vi "Add ItemIDs.vi"(8 "error in":errorcluster, 11 "Panel in":refnum<class "Panel.lvclass">) -> (0 "error out":errorcluster, 3 "Panel out":refnum<class "Panel.lvclass">)   [LabVIEW 2021]
uses:
  <vilib>/OPCUA/controls/Data Type.ctl
  <vilib>/OPCUA/NI OPC UA Server.lvlib
  Panel.lvclass
  C:/GitHub/SM EOL OPC Server AF/Station/Station Actor/Station.lvclass
  C:/Program Files/National Instruments/LabVIEW 2021/vi.lib/ActorFramework/Actor/Actor.lvclass
  C:/GitHub/SM EOL OPC Server AF/Station Panel/Station Panel Actor/Panel.lvclass
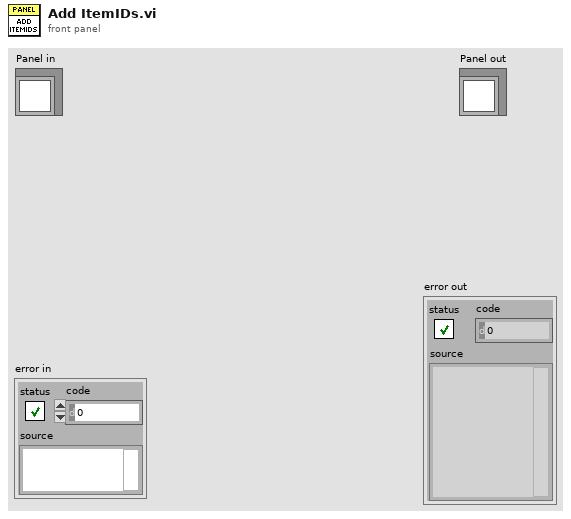
[diagram p1: front panel]
types:
  T1 = typedef "Data Type.ctl" = u16
  T2 = cluster{"name":string, "data type":T1, "access level":u16, "description":string}
  T3 = typedef "NodeId.ctl" = string
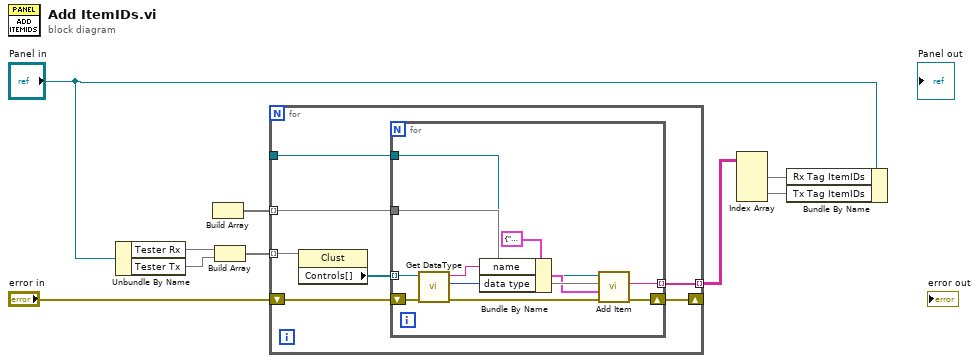
[diagram p0: block diagram]
diagram:
  n1 = Unbundle By Name("Panel in") -> ("Tester Rx"=w9, "Tester Tx"=w8)
  n2 = Build Array() -> (w2:void[])  [unwired: 2 in]
  n3 = Build Array(w9, w8) -> (w7:void[])
  n4 = for {
    tunnel: w7 -> [w14] mode=indexing
    tunnel: w2 -> [w13] mode=indexing
    tunnel: [w12] -> w5 mode=indexing
    shift-right: [w15] -> _
    shift-left: "error in" -> [w16]
    tunnel: _ -> [w10]
    n5 = property class="Clust"(reference=w14) -> ("Controls[]"=w11:refnum<vi>[])  [unwired: 1 in, 2 out]
    n6 = for {
      tunnel: w13 -> [w27]
      shift-right: [w26] -> w15
      shift-left: w16 -> [w21]
      tunnel: [w25] -> w12 mode=indexing
      tunnel: w11 -> [w22] mode=indexing
      tunnel: w10 -> [w17]
      n7 = call "Get DataType.vi"("error in (no error)"=w21, "reference"=w22) -> ("error out"=w19:errorcluster, "data type"=w18:T1, "Name"=w20:string)  [unwired: 7 in]
      n8 = Bundle By Name(cluster=T2 {"name"="", "data type"=1, "access level"=3, "description"=""} ("item"), "name"=w20, "data type"=w18) -> (w23:T2)
      n9 = call <vilib>:"Add Item.vi"("error in (no error)"=w19, "item"=w23, "parent folder node ID"=w27, "OPC UA server refnum in"=w17) -> ("error out"=w26:errorcluster, "item node ID"=w25:T3)  [unwired: 3 in, 2 out]
    }
  }
  n10 = Index Array(array=w5) -> (element #1=w4:T3[], element #2=w3:T3[])  [unwired: 4 in]
  n11 = Bundle By Name(cluster="Panel in", "Rx Tag ItemIDs"=w4, "Tx Tag ItemIDs"=w3) -> ()  [unwired: 1 out]
